vi "Test Data Conversion.vi"() -> ()   [LabVIEW 2019]
uses:
  src/LV-Data/Typedefs/Map Variant--map.ctl
  src/LV-Data/Typedefs/Dictionary--cluster.ctl
  d4e00cda-4e87-475a-9ac5-d9e4d4febcd8.vi
  b2b93d2e-0f75-4339-9965-6d089316595d.vi
  ee9872cd-08cb-463d-a526-4a2a65f3865f.vi
  ac946e30-71e5-44ba-80eb-c6018775c2f6.vi
  eba62c78-6134-4818-8f80-6934956bf520.vi
  35624f98-061d-41f6-bac3-4dadba41fd8c.vi
  8d87721e-5ac7-438b-b6ea-3a9496e7f386.vi
  b2e13f2b-f11a-4e67-8d8d-d6b785dda5d1.vi
  ee9872cd-08cb-463d-a526-4a2a65f3865f.vi/ecb17a1d-7eb0-4816-9ea9-fb6c805c284c.vi
  ac946e30-71e5-44ba-80eb-c6018775c2f6.vi/a1faece5-1cf7-40b8-b7e8-84859645c914.vi
  eba62c78-6134-4818-8f80-6934956bf520.vi/009dfa3b-8732-493e-8b3e-3c978875f984.vi
  eba62c78-6134-4818-8f80-6934956bf520.vi/8256e227-9b1a-43a9-8b6a-3cc1b0b1a82d.vi
  35624f98-061d-41f6-bac3-4dadba41fd8c.vi/428f5441-9cd4-4da4-ab8a-2b7aaf6bd19d.vi
  35624f98-061d-41f6-bac3-4dadba41fd8c.vi/26b40515-ff3d-4641-80e3-830eea05c610.vi
  8d87721e-5ac7-438b-b6ea-3a9496e7f386.vi/0af1b6d1-50c9-4fae-92cc-2c71bc32f23b.vi
  b2e13f2b-f11a-4e67-8d8d-d6b785dda5d1.vi/1cb9e1ca-6222-4b50-a6e9-c9c345a8e4b6.vi
  <vilib>/AdvancedString/1D String Array to Delimited String.vi
  src/LV-Data.ITX/private/Variant to ITX Wave.vi
  src/LV-Data.ITX/private/Commands to ITX.vi
  src/LV-Data.ITX/private/Notes to ITX.vi
  src/LV-Data/LV-Data.lvclass
panel:
  out "error out":errorcluster
  in  "folder":path
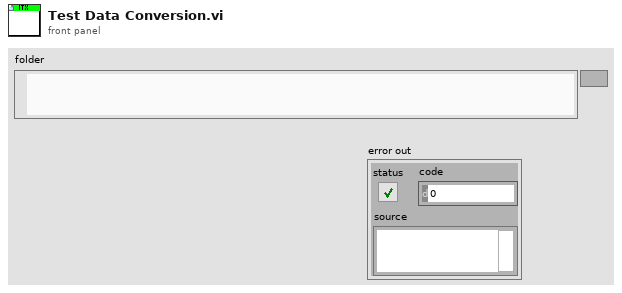
[diagram p1: front panel]
types:
  T1 = typedef "LV-Data.lvclass/Dictionary--cluster.ctl" = cluster{"key":string, "value":variant}
  T2 = typedef "LV-Data.lvclass/Map Variant--map.ctl" = map{string, variant}
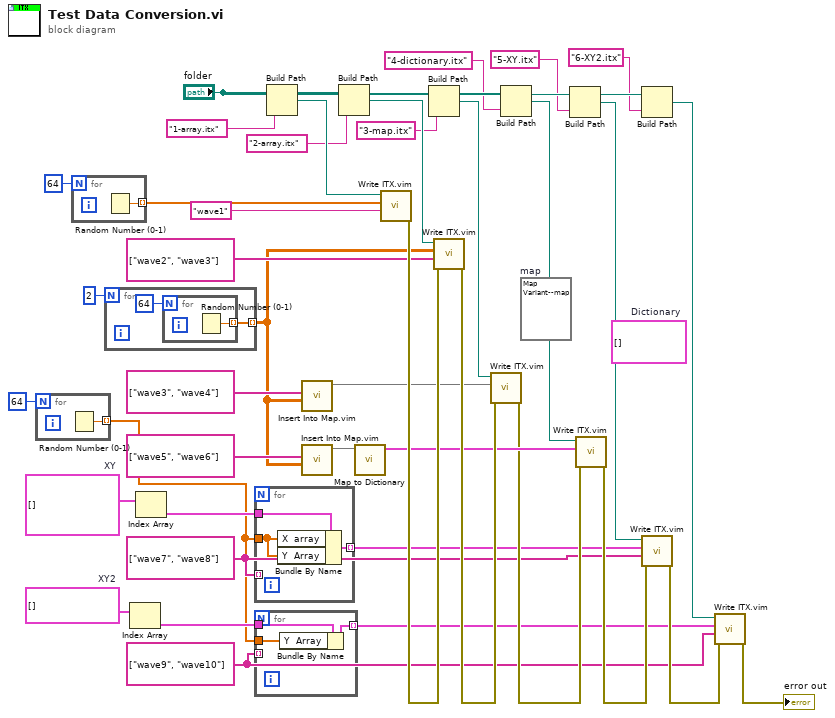
[diagram p0: block diagram]
diagram:
  w11 = string[] ["wave9", "wave10"]
  w10 = string[] ["wave7", "wave8"]
  (unwired) T1[] []  # Dictionary
  (unwired) T2 {}  # map
  w18 = cluster{"X  array":dbl[], "Y  Array":dbl[]}[] []  # XY
  w17 = cluster{"Y  Array":dbl[]}[] []  # XY2
  n1 = for {
    N: 64 -> [_]
    tunnel: [w41] -> w6 mode=indexing
    n2 = Random Number (0-1)() -> (number: 0 to 1=w41:dbl)
  }
  n3 = for {
    N: 64 -> [_]
    tunnel: [w42] -> w8 mode=indexing
    n4 = Random Number (0-1)() -> (number: 0 to 1=w42:dbl)
  }
  n5 = for {
    N: 2 -> [_]
    tunnel: [w43] -> w20 mode=indexing
    n6 = for {
      N: 64 -> [_]
      tunnel: [w45] -> w43 mode=indexing
      n7 = Random Number (0-1)() -> (number: 0 to 1=w45:dbl)
    }
  }
  n8 = Index Array(array=w17) -> (element=w16:cluster{"Y  Array":dbl[]})  [unwired: 1 in]
  n9 = Index Array(array=w18) -> (element=w15:cluster{"X  array":dbl[], "Y  Array":dbl[]})  [unwired: 1 in]
  n10 = for {
    tunnel: w15 -> [w48]
    tunnel: [w47] -> w13 mode=indexing
    tunnel: w10 -> [_] mode=indexing
    tunnel: w6 -> [w46]
    n11 = Bundle By Name(cluster=w48, "X  array"=w46, "Y  Array"=w46) -> (w47:cluster{"X  array":dbl[], "Y  Array":dbl[]})
  }
  n12 = for {
    tunnel: w16 -> [w51]
    tunnel: [w50] -> w14 mode=indexing
    tunnel: w11 -> [_] mode=indexing
    tunnel: w6 -> [w49]
    n13 = Bundle By Name(cluster=w51, "Y  Array"=w49) -> (w50:cluster{"Y  Array":dbl[]})
  }
  n14 = Build Path(base path="folder", name or relative path="1-array.itx") -> (appended path=w31:path)
  n15 = call "Insert Into Map.vim"("value"=w20, "key"=string[] ["wave3", "wave4"]) -> ("map out"=w7:T2)  [unwired: 8 in, 1 out]
  n16 = call "Insert Into Map.vim"("value"=w20, "key"=string[] ["wave5", "wave6"]) -> ("map out"=w19:T2)  [unwired: 8 in, 1 out]
  n17 = Build Path(base path="folder", name or relative path="2-array.itx") -> (appended path=w30:path)
  n18 = call "Map to Dictionary.vi"("map"=w19) -> ("Data (Dictionary)"=w35:T1[])  [unwired: 9 in, 1 out]
  n19 = call "Write ITX.vim"("wavename"="wave1", "values"=w8, "filename"=w31) -> ("error out"=w39:errorcluster)  [unwired: 6 in, 2 out]
  n20 = Build Path(base path="folder", name or relative path="3-map.itx") -> (appended path=w28:path)
  n21 = call "Write ITX.vim"("error in"=w39, "wavename"=string[] ["wave2", "wave3"], "values"=w20, "filename"=w30) -> ("error out"=w36:errorcluster)  [unwired: 5 in, 2 out]
  n22 = call "Write ITX.vim"("error in"=w36, "values"=w7, "filename"=w28) -> ("error out"=w34:errorcluster)  [unwired: 6 in, 2 out]
  n23 = Build Path(base path="folder", name or relative path="4-dictionary.itx") -> (appended path=w27:path)
  n24 = Build Path(base path="folder", name or relative path="5-XY.itx") -> (appended path=w26:path)
  n25 = call "Write ITX.vim"("error in"=w34, "values"=w35, "filename"=w27) -> ("error out"=w33:errorcluster)  [unwired: 6 in, 2 out]
  n26 = Build Path(base path="folder", name or relative path="6-XY2.itx") -> (appended path=w25:path)
  n27 = call "Write ITX.vim"("error in"=w33, "wavename"=w10, "values"=w13, "filename"=w26) -> ("error out"=w32:errorcluster)  [unwired: 5 in, 2 out]
  n28 = call "Write ITX.vim"("error in"=w32, "wavename"=w11, "values"=w14, "filename"=w25) -> ("error out"=→"error out":errorcluster)  [unwired: 5 in, 2 out]
